vi "SQL.PathListFilter.vi"(8 "错误输入":errorcluster, 9 "筛选条件":string, 10 "CMD":enum16{"筛选L1类路径(结果数据)", "筛选L2类路径(测试数据)"}(ring), 11 "Folder Path":path caption="文件夹路径") -> (0 "错误输出":errorcluster, 3 "PathList_Output":path[](array[path]))   [LabVIEW 2012, in "Lib_UEL.ATE.lvlib" / "Lib_SQL.lvlib"]
uses:
  <vilib>/regexp/Match Regular Expression.xnode
  Lib_SQL.lvlib
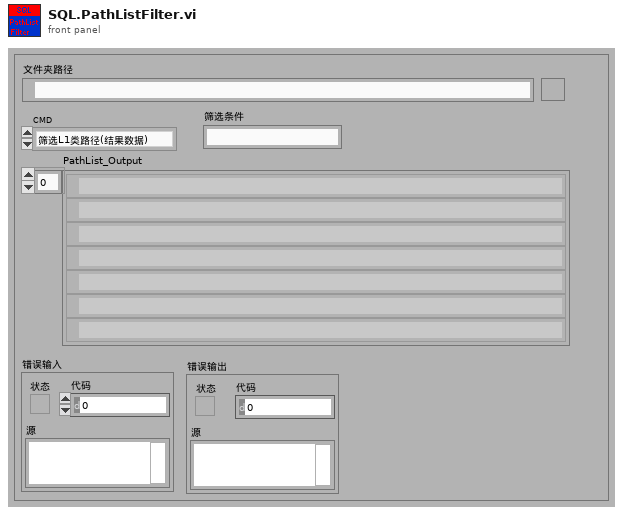
[diagram p1: front panel]
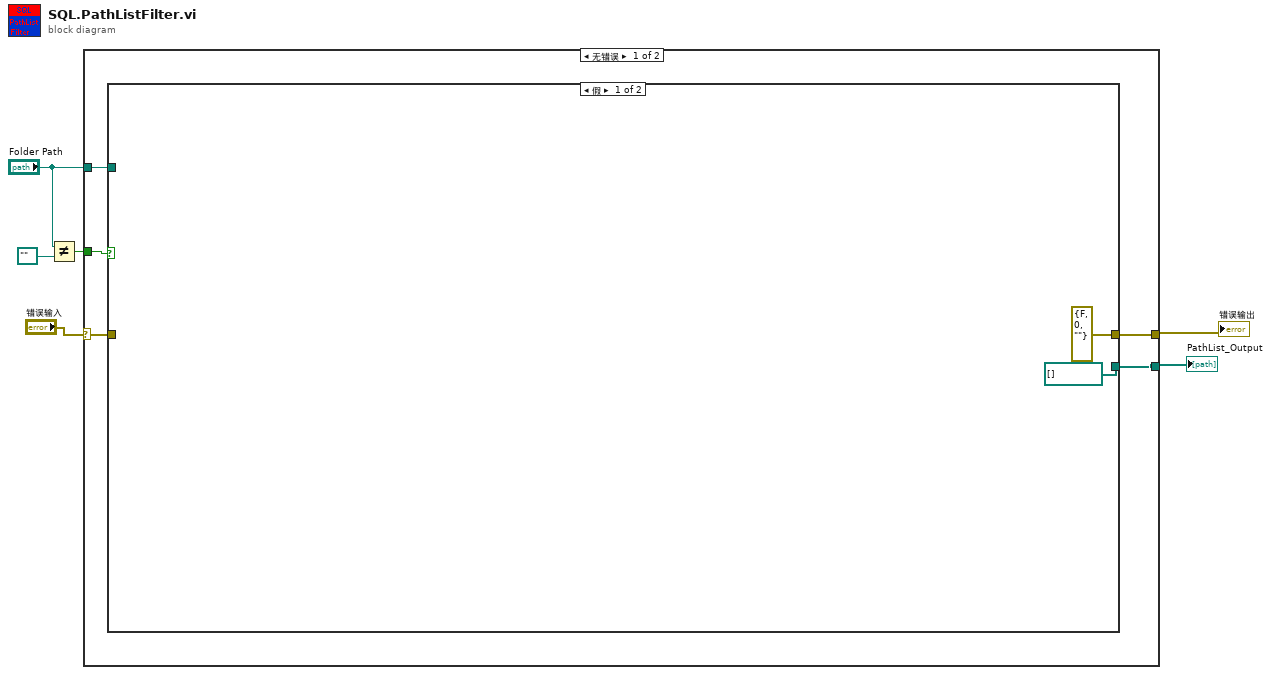
[diagram p0: block diagram]
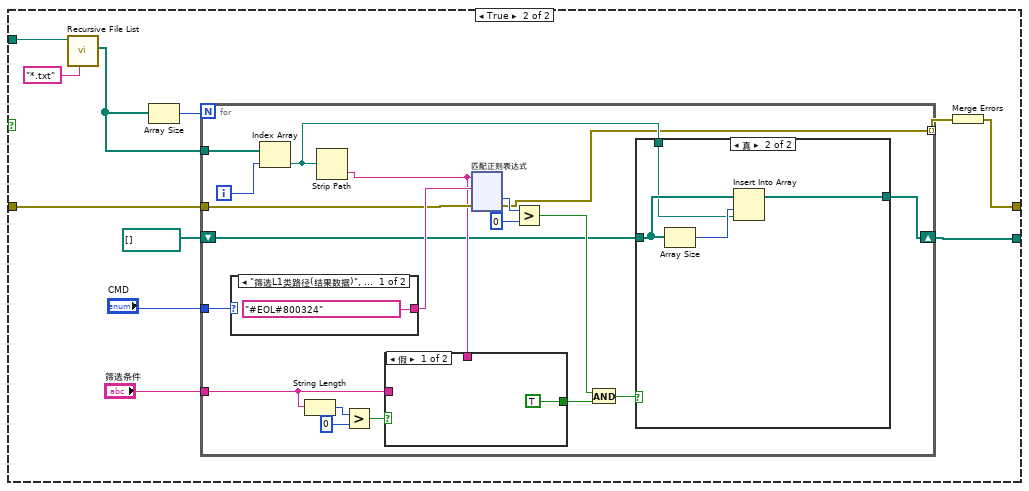
[diagram p2: hidden frame]
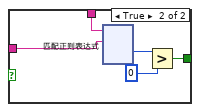
[diagram p4: hidden frame]
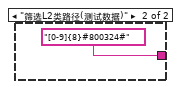
[diagram p5: hidden frame]
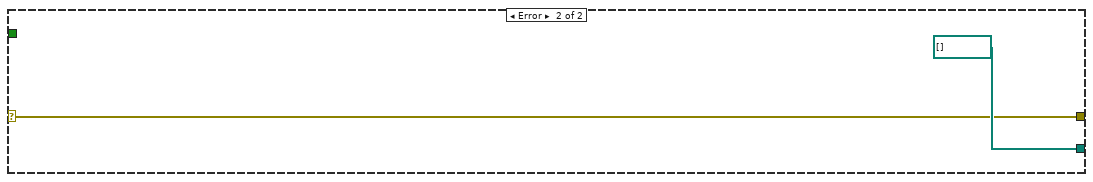
[diagram p6: hidden frame]
diagram:
  n1 = Not Equal?(x="Folder Path", y=path "") -> (x != y?=w1:bool)
  n2 = case shown="无错误" "错误输入" {
    selector: "错误输入" -> [w10 w279]
    tunnel: [w11 path[] [] ("PathList")] -> w6
    tunnel: [w9 w279] -> w4
    tunnel: "Folder Path" -> [w8 _]
    tunnel: w1 -> [w7 _]
    frame No Error {
      n3 = case shown="假" w7 {
        tunnel: [path[] [] ("PathList") w21] -> w11
        tunnel: w10 -> [_ w20]
        tunnel: [errorcluster {"status"=FALSE, "code"=0, "source"=""} ("error out") w17] -> w9
        tunnel: w8 -> [_ w15]
        frame False {
        }
        frame True {
          n4 = call <vilib>:"Recursive File List.vi"("pattern"="*.txt", "Folder Path"=w15) -> ("All Files in Dir"=w14:path[])  [unwired: 5 in, 4 out]
          n5 = Array Size(array=w14) -> (size(s)=w24:i32)
          n6 = for {
            N: w24 -> [_]
            shift-right: [w26] -> w21
            shift-left: path[] [] ("PathList") -> [w28]
            tunnel: w14 -> [w43]
            tunnel: "CMD" -> [w41]
            tunnel: w20 -> [w39]
            tunnel: "筛选条件" -> [w35]
            tunnel: [w25] -> w18 mode=indexing
            i -> [w42]
            n7 = case shown="\"筛选L1类路径(结果数据)\", 默认" w41 {
              tunnel: ["#EOL#800324" ("正则表达式") "[0-9]{8}#800324#" ("正则表达式")] -> w40
              frame "筛选L1类路径(结果数据)", Default {
              }
              frame "筛选L2类路径(测试数据)" {
              }
            }
            n8 = Index Array(array=w43, index=w42) -> (element=w27:path)
            n9 = String Length(string=w35) -> (length=w34:i32)
            n10 = Strip Path(path=w27) -> (name=w36:string)  [unwired: 1 out]
            n11 = Greater?(x=w34, y=0) -> (0:w32:bool)
            n12 = case shown="假" w32 {
              tunnel: w36 -> [_ w54]
              tunnel: w35 -> [_ w51]
              tunnel: [TRUE w50] -> w31
              frame False {
              }
              frame True {
                n13 = xnode "匹配正则表达式"("输入字符串"=w54, "正则表达式"=w51) -> ("匹配后偏移量"=w53:i32)  [unwired: 4 in, 4 out]
                n14 = Greater?(x=w53, y=0) -> (0:w50:bool)
              }
            }
            n15 = xnode "匹配正则表达式"("输入字符串"=w36, "正则表达式"=w40, "错误输入"=w39) -> ("匹配后偏移量"=w38:i32, "错误输出"=w25:errorcluster)  [unwired: 3 in, 3 out]
            n16 = Greater?(x=w38, y=0) -> (0:w30:bool)
            n17 = And(x=w30, y=w31) -> (x .and. y?=w29:bool)
            n18 = case shown="真" w29 {
              tunnel: w28 -> [w44 w48]
              tunnel: w27 -> [_ w46]
              tunnel: [w44 w45] -> w26
              frame False {
              }
              frame True {
                n19 = Array Size(array=w48) -> (size(s)=w47:i32)
                n20 = Insert Into Array(array=w48, index=w47, new element=w46) -> (w45:path[])
              }
            }
          }
          n21 = Merge Errors(w18) -> (w17:errorcluster)
        }
      }
    }
    frame Error {
    }
  }
  "PathList_Output" <- w6
  "错误输出" <- w4
